vi "permutate.vi"(10 "PermutationsLimit":i32=100000, 11 "Input":string[](array[string])) -> (3 "Permutations":string[][](array[string]))   [LabVIEW 2014]
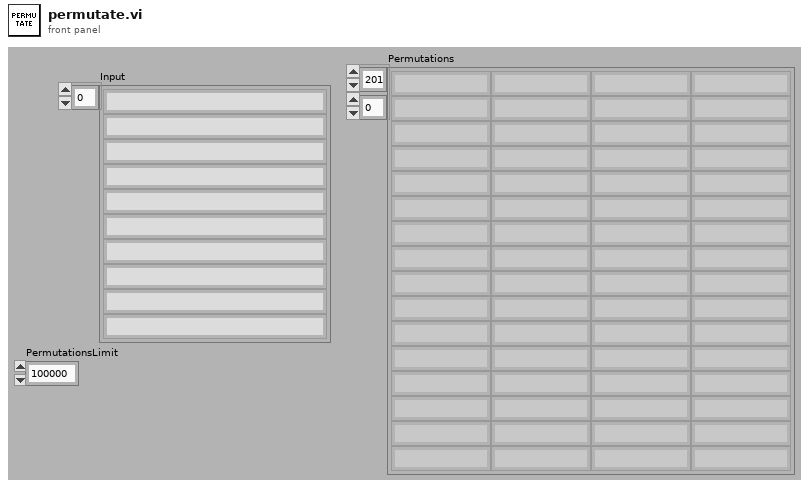
[diagram p1: front panel]
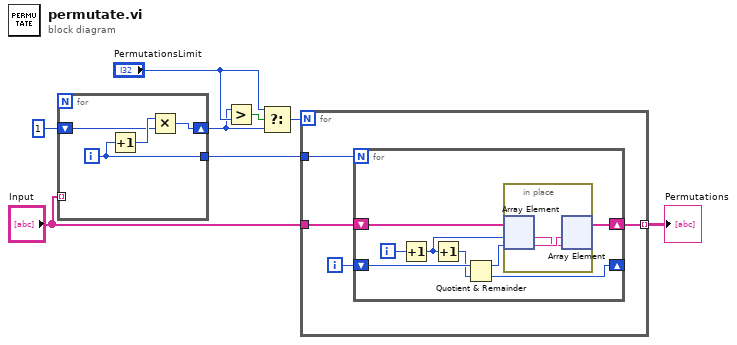
[diagram p0: block diagram]
diagram:
  n1 = for {
    shift-right: [w11] -> w2
    shift-left: 1 -> [w10]
    tunnel: "Input" -> [_] mode=indexing
    tunnel: [w9] -> w7
    i -> [w9]
    n2 = Increment(x=w9) -> (x+1=w12:i32)
    n3 = Multiply(x=w12, y=w10) -> (x*y=w11:i32)
  }
  n4 = Greater?(x=w2, y="PermutationsLimit") -> (0:w4:bool)
  n5 = Select(t="PermutationsLimit", s=w4, f=w2) -> (s? t:f=w1:i32)
  n6 = for {
    N: w1 -> [_]
    tunnel: w7 -> [w16]
    tunnel: "Input" -> [w15]
    tunnel: [w13] -> w5 mode=indexing
    i -> [w14]
    n7 = for "loop over j (2..length(s))" {
      N: w16 -> [_]
      shift-right: [w17] -> w13
      shift-left: w15 -> [w19]
      shift-right: [w22] -> _
      shift-left: w14 -> [w24]
      i -> [w23]
      n8 = Increment(x=w23) -> (x+1=w20:i32)
      n9 = Increment(x=w20) -> (x+1=w21:i32)
      n10 = Quotient & Remainder(x=w24, y=w21) -> (x-y*floor(x/y)=w18:i32, floor(x/y)=w22:i32)
      n11 = in-place {
        n12 = in-place-array #1(w19, w20, w18) -> (w25:string, w26:string)
        n13 = in-place-array #1(w26, w25) -> (w17:string[])  [unwired: 2 out]
      }
    }
  }
  "Permutations" <- w5
